vi "beginPassTo2ndStrikerPlay.vi"(8 "error in (no error)":errorcluster, 10 "Game":refnum<class "Game.lvclass">, 11 "PassTo2ndStriker in":refnum<class "PassTo2ndStriker.lvclass">) -> (0 "error out":errorcluster, 2 "result":bool, 3 "PassTo2ndStriker out":refnum<class "PassTo2ndStriker.lvclass">)   [LabVIEW 2023, in "PassTo2ndStriker.lvclass"]
uses:
  PassTo2ndStriker.lvclass
  Game_class/Game.lvclass
  Utilities_class/Utilities.lvclass
  Referee_class/command_interpreted.ctl
  Team_class/OffensivePlay.ctl
  Game_class/Game.lvclass/Game.ctl
  Referee_class/Referee.lvclass/Referee.ctl
  Team_class/Team.lvclass/Team.ctl
  Game_class/Read OffensiveTeam.vi
  Team_class/Read RobotRef.vi
  Team_class/Read OffensivePlay.vi
  Game_class/Read AllyRef.vi
  Game_class/Read Referee.vi
  Referee_class/Read command_interpreted.vi
  Ally_class/Ally.lvclass
  C:/Users/roboi/Downloads/VSS_AI-Larc2023/Team_class/Team.lvclass
  Referee_class/Referee.lvclass
  Robot_class/Robot.lvclass
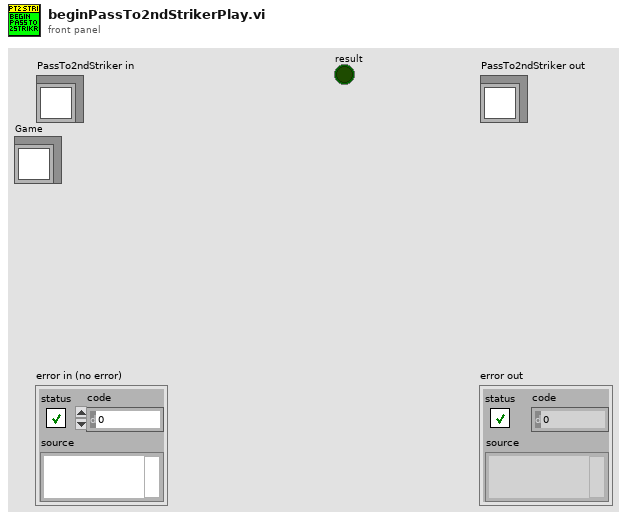
[diagram p1: front panel]
types:
  T1 = typedef "OffensivePlay.ctl" = enum16{"TableWithStriker", "TableWith2ndStrikerPlay", "PrepareDoublePass", "PrepareRollToPass", "SimplePass", "PreparePass", "PassToStriker", "BallOutOfField", "PassTo2ndStriker", "StopOffensive", "Prepare Penalty Enemy", "EnemyPossessionAtEnemyField", "EnemyPossesionAtOurField", "TestPlay", "PreparePenaltyAlly", "KickPenaltyAlly", "PrepareKickoffAlly", "PrepareKickoffEnemy", "IndirectEnemy", "DirectEnemy", "NormalGame", "DirectKick", "Pass", "Halt", "Timeout", "PassPlay", "PenaltyEnemy"}
  T2 = typedef "command_interpreted.ctl" = enum16{"Goal Ally", "Goal Enemy", "Ball Placement Enemy", "Ball Placement Ally", "Normal Half Time", "Extra Time  Break", "Extra Half Time", "None", "Post Game", "PKA Normal Start", "Prepare Kickoff Ally", "PKE Normal Start", "Prepare Kickoff Enemy", "Force Start", "Halt", "Timeout", "Prepare Penalty Ally", "Prepare Penalty Enemy", "PPA NormalStart", "PPE Normal Start", "Indirect Free Ally", "Direct Free Enemy", "Direct Free Ally", "Indirect Free Enemy", "Stop"}
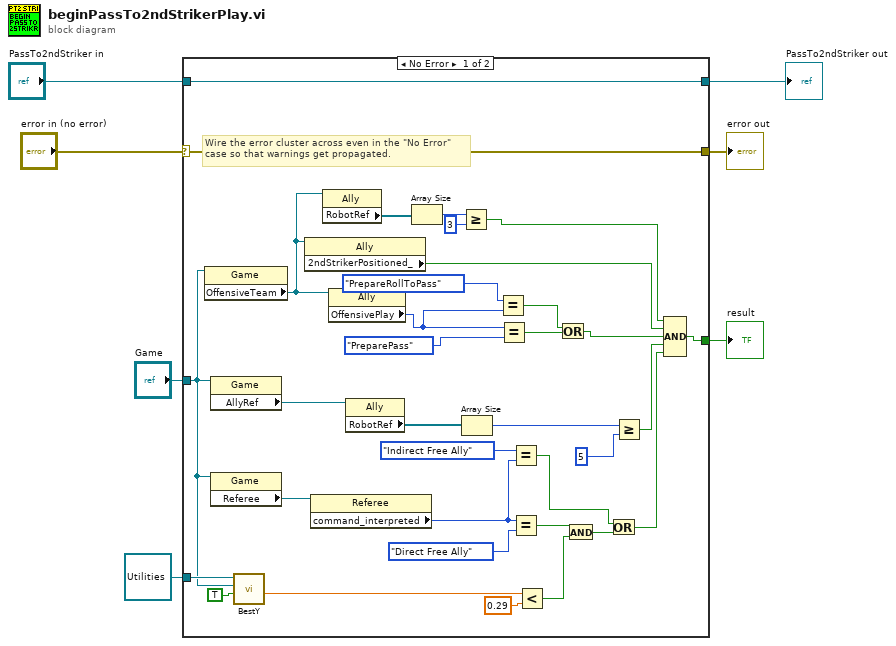
[diagram p0: block diagram]
diagram:
  n1 = case shown="No Error" "error in (no error)" {
    selector: "error in (no error)" -> [w40 w43]
    tunnel: [w40 w43] -> w6
    tunnel: [w41 w42] -> w4
    tunnel: "PassTo2ndStriker in" -> [w41 w42]
    tunnel: "Game" -> [w25 _]
    tunnel: refnum<class "Utilities.lvclass"> refnum ("Utilities.lvclass") -> [w31 _]
    tunnel: [w24 _] -> w1
    frame No Error {
      # "Wire the error cluster across even in the \"No Error\"\ncase so that warnings get propagated."
      n2 = property class="Game"(reference=w25) -> ("OffensiveTeam"=w12:refnum<class "Ally.lvclass">)  [unwired: 1 in, 2 out]
      n3 = property class="Game"(reference=w25) -> ("AllyRef"=w30:refnum<class "Ally.lvclass">)  [unwired: 1 in, 2 out]
      n4 = property class="Game"(reference=w25) -> ("Referee"=w39:refnum<class "Referee.lvclass">)  [unwired: 1 in, 2 out]
      n5 = call "BestY.vi"("Utilities in"=w31, "Game"=w25, "inimigos"=TRUE) -> ("Gap kick"=w33:dbl)  [unwired: 2 in, 4 out]
      n6 = property class="Ally"(reference=w12) -> ("2ndStrikerPositioned_"=w27:bool)  [unwired: 1 in, 2 out]
      n7 = property class="Referee"(reference=w39) -> ("command_interpreted"=w37:T2)  [unwired: 1 in, 2 out]
      n8 = property class="Ally"(reference=w12) -> ("RobotRef"=w11:refnum<class "Robot.lvclass">[])  [unwired: 1 in, 2 out]
      n9 = property class="Ally"(reference=w12) -> ("OffensivePlay"=w15:T1)  [unwired: 1 in, 2 out]
      n10 = property class="Ally"(reference=w30) -> ("RobotRef"=w29:refnum<class "Robot.lvclass">[])  [unwired: 1 in, 2 out]
      n11 = Array Size(array=w11) -> (size(s)=w10:i32)
      n12 = Greater Or Equal?(x=w10, y=3) -> (x >= y?=w8:bool)
      n13 = Array Size(array=w29) -> (size(s)=w28:i32)
      n14 = Equal?(x=OffensivePlay."PrepareRollToPass" ("OffensivePlay"), y=w15) -> (x = y?=w13:bool)
      n15 = Equal?(x=w15, y=OffensivePlay."PreparePass" ("OffensivePlay")) -> (x = y?=w17:bool)
      n16 = Equal?(x=command_interpreted."Indirect Free Ally" ("command_interpreted"), y=w37) -> (x = y?=w20:bool)
      n17 = Equal?(x=w37, y=command_interpreted."Direct Free Ally" ("command_interpreted")) -> (x = y?=w22:bool)
      n18 = Less?(x=w33, y=0.29 ("Gap kick")) -> (x < y?=w32:bool)
      n19 = Or(x=w13, y=w17) -> (x .or. y?=w16:bool)
      n20 = And(x=w22, y=w32) -> (x .and. y?=w21:bool)
      n21 = Or(x=w20, y=w21) -> (x .or. y?=w19:bool)
      n22 = Greater Or Equal?(x=w28, y=5) -> (x >= y?=w26:bool)
      n23 = Compound Arithmetic op=AND(w8, w27, w16, w26, w19) -> (w24:bool)
    }
    frame Error {
    }
  }
  "error out" <- w6
  "PassTo2ndStriker out" <- w4
  "result" <- w1
